vi "Falling Edge Detector.vi"(1 "Input":bool) -> (0 "Falling Edge Detected":bool)   [LabVIEW 2015]
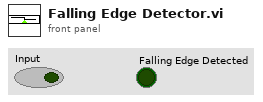
[diagram p1: front panel]
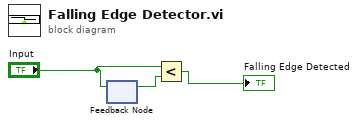
[diagram p0: block diagram]
diagram:
  n1 = feedback #1() -> (w2:bool)  [unwired: 1 in]
  n2 = feedback-in #1("Input") -> ()
  n3 = Less?(x="Input", y=w2) -> (x < y?=→"Falling Edge Detected":bool)
